vi "zad5.vi"() -> ()   [LabVIEW 2017]
panel:
  in  "stop":bool
  in  "Działanie":T1(radio)=enum."Dzielenie"
  out "Wynik":dbl
  in  "B":dbl
  in  "A":dbl
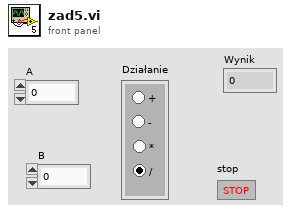
[diagram p1: front panel]
types:
  T1 = enum32{"No Selection", "Dodawanie", "Mnożenie", "Dzielenie", "Odejmowanie"}
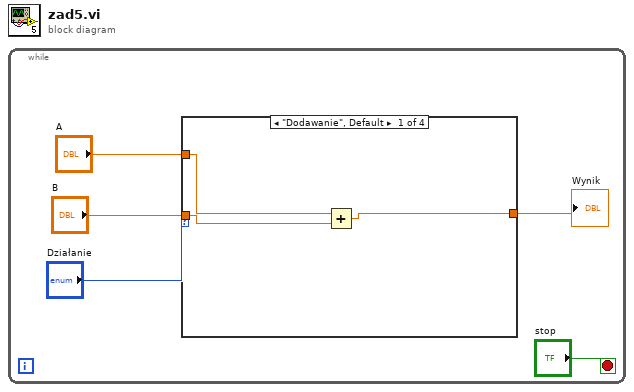
[diagram p0: block diagram]
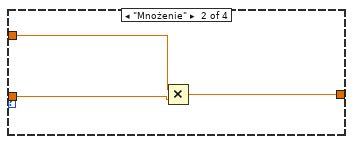
[diagram p2: hidden frame]
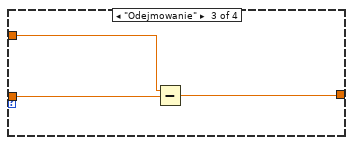
[diagram p3: hidden frame]
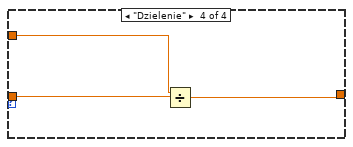
[diagram p4: hidden frame]
diagram:
  n1 = while {
    stop <- "stop" stop-if-true
    n2 = case shown="\"Dodawanie\", Default" "Działanie" {
      tunnel: "A" -> [w8 w11 w14 w17]
      tunnel: "B" -> [w6 w10 w13 w15]
      tunnel: [w7 w9 w12 w16] -> w1
      frame "Dodawanie", Default {
        n3 = Add(x=w8, y=w6) -> (x+y=w7:dbl)
      }
      frame "Mnożenie" {
        n4 = Multiply(x=w11, y=w10) -> (x*y=w9:dbl)
      }
      frame "Odejmowanie" {
        n5 = Subtract(x=w14, y=w13) -> (x-y=w12:dbl)
      }
      frame "Dzielenie" {
        n6 = Divide(x=w17, y=w15) -> (x/y=w16:dbl)
      }
    }
    "Wynik" <- w1
  }
